vi "Compare and Append Cell.vi"(8 "Schedule Cell B in":refnum<class "Schedule Cell.lvclass">, 11 "Optimiser Cell A in":refnum<class "Optimiser Cell.lvclass">) -> (0 "Schedule Cell B out":refnum<class "Schedule Cell.lvclass">, 2 "Cell Updated":bool, 3 "Optimiser Cell A out":refnum<class "Optimiser Cell.lvclass">)   [LabVIEW 2020, in "Run Utilities.lvlib" / "Optimiser Cell.lvclass"]
doc: "Compare two cells. If they have the same script the function modifies the cell A (increases number of repetitions) and returns true. Otherwise, the function returns unmodified cells and false."
uses:
  Optimiser Cell.lvclass
  C:/Users/marco/Documents/GitHub_Lab/TALOS/talos/Run Utilities/Cell/Schedule Cell.lvclass
  Cell/Schedule Cell.lvclass
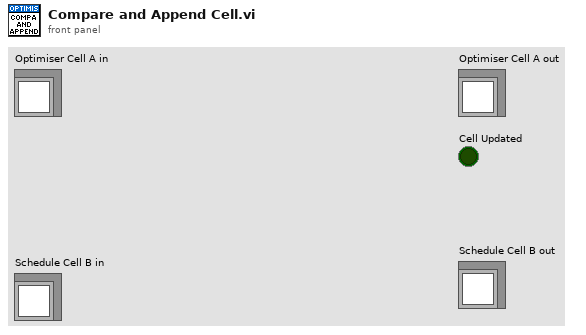
[diagram p1: front panel]
types:
  T1 = typedef "Run Utilities.lvlib/Optimiser Cell.lvclass/Optimiser Results.ctl" = cluster{"Array of Parameters":T2[], "Target":string}
  T2 = typedef "Analysis Framework.lvclass/Name with value pair.ctl" = cluster{"Name":string, "Value":string}
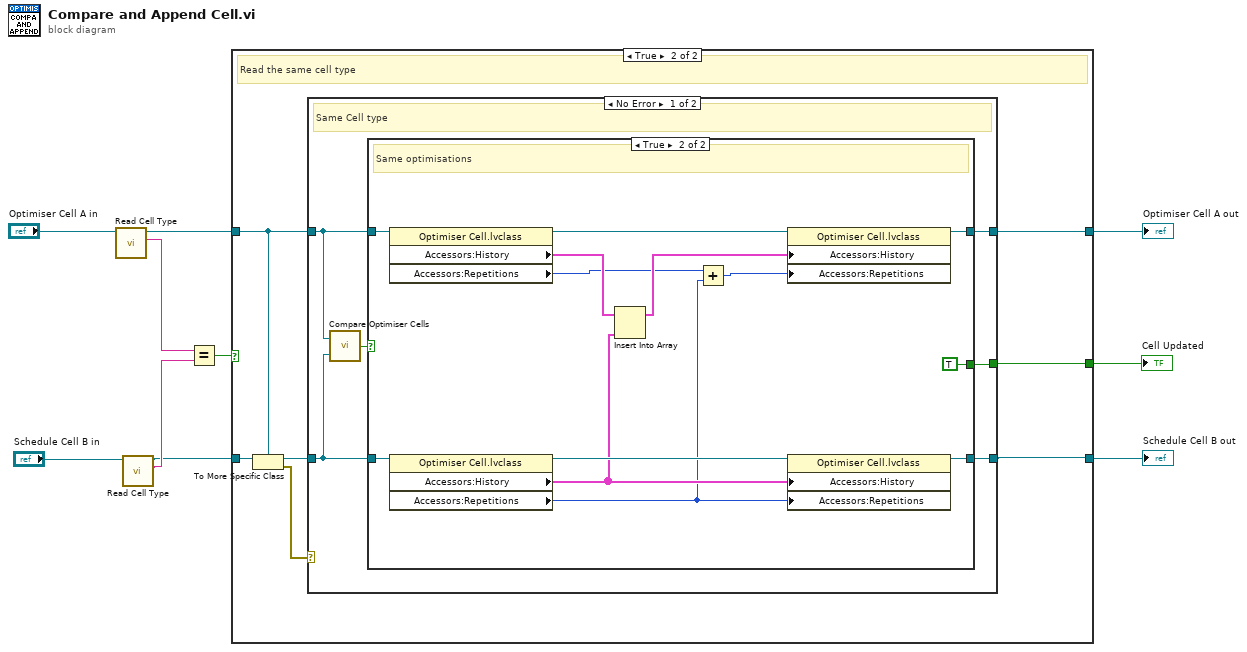
[diagram p0: block diagram]
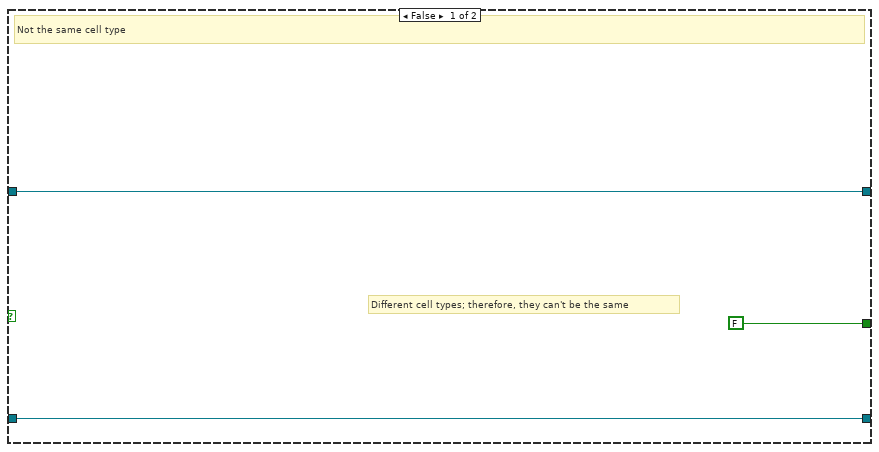
[diagram p2: hidden frame]
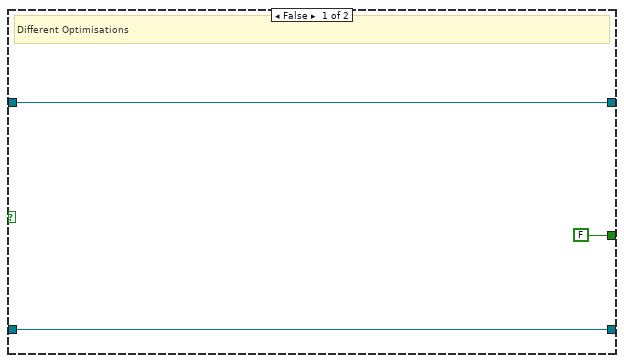
[diagram p3: hidden frame]
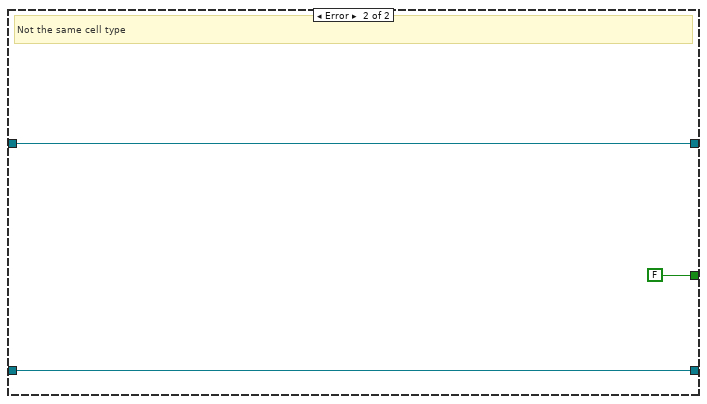
[diagram p4: hidden frame]
diagram:
  n1 = call-dynamic "Read Cell Type.vi"("Optimiser Cell in"="Optimiser Cell A in") -> ("Cell Type"=w6:string, "Optimiser Cell out"=w7:refnum<class "Optimiser Cell.lvclass">)  [unwired: 8 in, 1 out]
  n2 = call-dynamic "Read Cell Type.vi"("Schedule Cell in"="Schedule Cell B in") -> ("Cell Type"=w9:string, "Schedule Cell out"=w8:refnum<class "Schedule Cell.lvclass">)  [unwired: 8 in, 1 out]
  n3 = Equal?(x=w6, y=w9) -> (x = y?=w10:bool)
  n4 = case shown="True" w10 {
    tunnel: w7 -> [w12 w18]
    tunnel: [w12 w15] -> w5
    tunnel: w8 -> [w13 w20]
    tunnel: [w13 w14] -> w4
    tunnel: [FALSE w16] -> w3
    frame False {
      # "Different cell types; therefore, they can't be the same"
      # "Not the same cell type"
    }
    frame True {
      # "Read the same cell type"
      n5 = To More Specific Class(target class=w18, reference=w20) -> (specific class reference=w17:refnum<class "Optimiser Cell.lvclass">, error out=w19:errorcluster)  [unwired: 1 in]
      n6 = case shown="No Error" w19 {
        tunnel: [w26 w45] -> w15
        tunnel: w18 -> [w25 w45]
        tunnel: w17 -> [w24 w44]
        tunnel: [w22 w44] -> w14
        tunnel: [w21 FALSE] -> w16
        frame No Error {
          # "Same Cell type"
          n7 = call "Compare Optimiser Cells.vi"("Optimieser Cell B"=w24, "Optimieser Cell A"=w25) -> ("Equal"=w23:bool)
          n8 = case shown="True" w23 {
            tunnel: [w29 w40] -> w26
            tunnel: w25 -> [w29 w41]
            tunnel: w24 -> [w28 w36]
            tunnel: [w28 w35] -> w22
            tunnel: [FALSE TRUE] -> w21
            frame False {
              # "Different Optimisations"
            }
            frame True {
              # "Same optimisations"
              n9 = property class="Optimiser Cell.lvclass"(reference=w41) -> (reference out=w39:refnum<class "Optimiser Cell.lvclass">, "Accessors:History"=w38:T1[], "Accessors:Repetitions"=w32:u32)  [unwired: 1 in, 1 out]
              n10 = property class="Optimiser Cell.lvclass"(reference=w36) -> (reference out=w34:refnum<class "Optimiser Cell.lvclass">, "Accessors:History"=w33:T1[], "Accessors:Repetitions"=w30:u32)  [unwired: 1 in, 1 out]
              n11 = Insert Into Array(array=w38, new element=w33) -> (w37:T1[])  [unwired: 1 in]
              n12 = Add(x=w32, y=w30) -> (x+y=w31:u32)
              n13 = property class="Optimiser Cell.lvclass"(reference=w39, "Accessors:History"=w37, "Accessors:Repetitions"=w31) -> (reference out=w40:refnum<class "Optimiser Cell.lvclass">)  [unwired: 1 in, 1 out]
              n14 = property class="Optimiser Cell.lvclass"(reference=w34, "Accessors:History"=w33, "Accessors:Repetitions"=w30) -> (reference out=w35:refnum<class "Optimiser Cell.lvclass">)  [unwired: 1 in, 1 out]
            }
          }
        }
        frame Error {
          # "Not the same cell type"
        }
      }
    }
  }
  "Optimiser Cell A out" <- w5
  "Cell Updated" <- w3
  "Schedule Cell B out" <- w4
